vi "Actor Core.vi"(8 "error in":errorcluster, 11 "HIJ Vision Camera App Dialog in":refnum<class "HIJ Vision Camera App Dialog.lvclass">) -> (0 "error out":errorcluster, 3 "Actor out":refnum<class "Actor.lvclass">)   [LabVIEW 2014, in "HIJ Vision Camera App Dialog.lvlib" / "HIJ Vision Camera App Dialog.lvclass"]
doc: "(<B>Filename</B>: Actor Framework.lvlib:Actor.lvclass:Actor Core.vi)\n\nReceives messages to the actor, reacts to them, and initiates any error handling that may shut the actor down.\n\nDescendant classes may override this VI to append parallel tasks for the actor to complete while it handles messages. Overrides use the Call Parent Method node."
uses:
  HIJ Vision Camera App Dialog.lvclass
  <vilib>/ActorFramework/Actor/Actor.lvclass
  <vilib>/userdefined/High Color/IMAQdx.ctl
  Shared Code/Viewable Actor/ViewableActor/ViewableActor.lvclass/ViewableActor.ctl
  HIJ Vision Camera App Dialog.lvclass/HIJ Vision Camera App Dialog.ctl
  <vilib>/ActorFramework/Actor/Actor.lvclass/Actor.ctl
  <vilib>/ActorFramework/Message Enqueuer/Message Enqueuer.lvclass/Message Enqueuer.ctl
  HIJ Vision Camera App Dialog Messages/Update Data befor stop Msg/Update Data befor stop Msg.lvclass/Update Data befor stop Msg.ctl
  HIJ Vision Camera App/HIJ Vision Camera App Messages/Save Sequence Msg/Save Sequence Msg.lvclass/Save Sequence Msg.ctl
  HIJ Vision Application/HIJ Vision Application Messages/Write WorkDir Msg/Write WorkDir Msg.lvclass/Write WorkDir Msg.ctl
  HIJ Vision Camera App/HIJ Vision Camera App Messages/Write ConfigDir Msg/Write ConfigDir Msg.lvclass/Write ConfigDir Msg.ctl
  HIJ Vision Application/HIJ Vision Application Messages/Write Image Prefix Msg/Write Image Prefix Msg.lvclass/Write Image Prefix Msg.ctl
  HIJ Vision Camera App/HIJ Vision Camera App Messages/Start Aquisition Msg/Start Aquisition Msg.lvclass/Start Aquisition Msg.ctl
  HIJ Vision Camera App/HIJ Vision Camera App Messages/Change Camera Msg/Change Camera Msg.lvclass/Change Camera Msg.ctl
  Shared Code/Viewable Actor/ViewableActor/Write UI VI Ref.vi
  Read Camera Name.vi
  Read ConfigDir.vi
  Read Prefix.vi
  Read WorkDir.vi
  Read Acquire.vi
  <vilib>/ActorFramework/Message Enqueuer/Init from Existing Queue.vi
  <vilib>/ActorFramework/Message Enqueuer/Enqueue.vi
  <vilib>/ActorFramework/Message Priority Queue/Priority Enqueue.vi
  <vilib>/ActorFramework/Message Enqueuer/Message Enqueuer.lvclass
  HIJ Vision Camera App Dialog Messages/Update Data befor stop Msg/Update Data befor stop Msg.lvclass
  <vilib>/ActorFramework/Stop Msg/Stop Msg.lvclass
  HIJ Vision Camera App/HIJ Vision Camera App Messages/Save Sequence Msg/Save Sequence Msg.lvclass
  HIJ Vision Application/HIJ Vision Application Messages/Write WorkDir Msg/Write WorkDir Msg.lvclass
  HIJ Vision Camera App/HIJ Vision Camera App Messages/Write ConfigDir Msg/Write ConfigDir Msg.lvclass
  HIJ Vision Application/HIJ Vision Application Messages/Write Image Prefix Msg/Write Image Prefix Msg.lvclass
  HIJ Vision Camera App/HIJ Vision Camera App Messages/Stop Aquisition Msg/Stop Aquisition Msg.lvclass
  HIJ Vision Camera App/HIJ Vision Camera App Messages/Start Aquisition Msg/Start Aquisition Msg.lvclass
  HIJ Vision Camera App/HIJ Vision Camera App Messages/Change Camera Msg/Change Camera Msg.lvclass
  Shared Code/Viewable Actor/ViewableActor/ViewableActor.lvclass
panel:
  in  "Acquire":bool
  in  "stop":bool
  in  "Camera Name":T1="TestCam"
  in  "#to save":u16=10
  in  "Save Seq.":bool
  in  "Prefix":string
  out "Current Nr.":u16=10
  in  "WorkDir":path=path "C:/Users/user/Desktop/test/WorkDir"
  in  "ConfigDir":path=path "C:/Users/user/Desktop/test/ConfigDir"
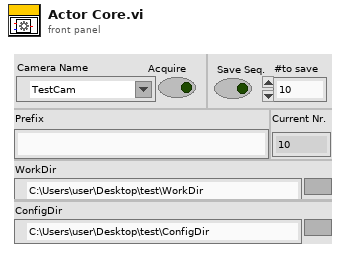
[diagram p1: front panel]
types:
  T1 = typedef "IMAQdx.ctl" = refnum<k21>
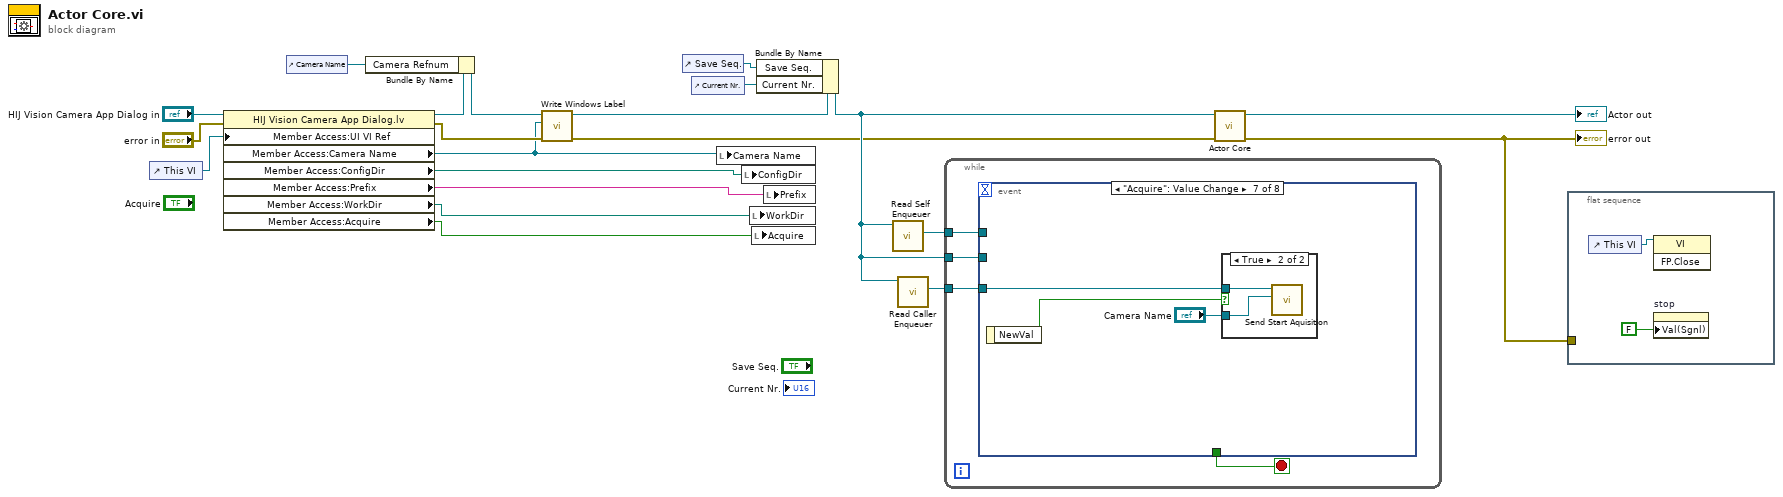
[diagram p0: block diagram]
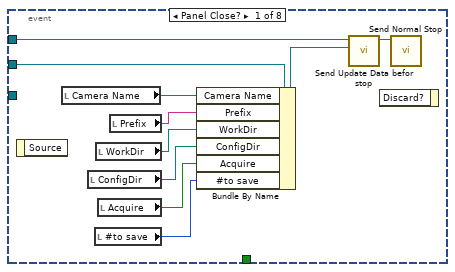
[diagram p2: hidden frame]
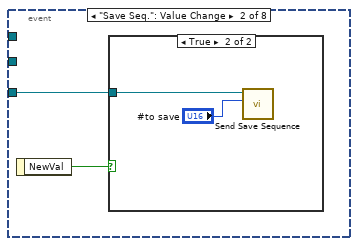
[diagram p3: hidden frame]
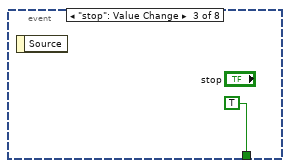
[diagram p5: hidden frame]
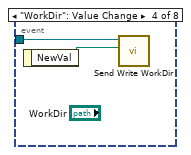
[diagram p6: hidden frame]
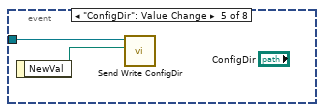
[diagram p7: hidden frame]
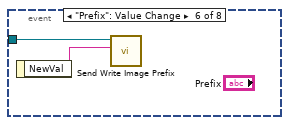
[diagram p8: hidden frame]
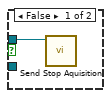
[diagram p9: hidden frame]
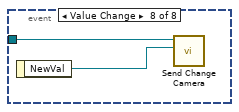
[diagram p10: hidden frame]
diagram:
  n1 = control-ref of="This VI"() -> (w17:refnum<vi>)
  n2 = property class="HIJ Vision Camera App Dialog.lv"(reference="HIJ Vision Camera App Dialog in", error in="error in", "Member Access:UI VI Ref"=w17) -> (reference out=w7:refnum<class "HIJ Vision Camera App Dialog.lvclass">, error out=w5:errorcluster, "Member Access:Camera Name"=w3:T1, "Member Access:ConfigDir"=w13:path, "Member Access:Prefix"=w12:string, "Member Access:WorkDir"=w14:path, "Member Access:Acquire"=w11:bool)
  n3 = control-ref of="Camera Name"() -> (w1:refnum<vi>)
  n4 = Bundle By Name(cluster=w7, "Camera Refnum"=w1) -> (w2:refnum<class "HIJ Vision Camera App Dialog.lvclass">)
  n5 = call-dynamic "Write Windows Label.vi"("error in (no error)"=w5, "Windows Label"=w3, "ViewableActor in"=w2) -> ("error out"=w4:errorcluster, "ViewableActor out"=w6:refnum<class "HIJ Vision Camera App Dialog.lvclass">)  [unwired: 7 in]
  n6 = control-ref of="Save Seq."() -> (w8:refnum<vi>)
  n7 = control-ref of="Current Nr."() -> (w9:refnum<vi>)
  n8 = local write "Camera Name"(w3) -> ()
  n9 = local write "ConfigDir"(w13) -> ()
  n10 = local write "WorkDir"(w14) -> ()
  n11 = local write "Acquire"(w11) -> ()
  n12 = Bundle By Name(cluster=w6, "Save Seq."=w8, "Current Nr."=w9) -> (w10:refnum<class "HIJ Vision Camera App Dialog.lvclass">)
  n13 = local write "Prefix"(w12) -> ()
  n14 = call <vilib>:"Read Self Enqueuer.vi"("Actor"=w10) -> ("Self Enqueuer"=w20:refnum<class "Message Enqueuer.lvclass">)  [unwired: 10 in]
  n15 = call <vilib>:"Read Caller Enqueuer.vi"("Actor"=w10) -> ("Caller Enqueuer"=w15:refnum<class "Message Enqueuer.lvclass">)  [unwired: 10 in]
  n16 = while {
    tunnel: w20 -> [w25]
    tunnel: w15 -> [w23]
    tunnel: w10 -> [w22]
    stop <- w24 stop-if-true
    n17 = event shown="[6] \"Acquire\": Value Change" {
      selector: _ -> [_ _ _ _ _ _ _ _]
      dyn-events: _ -> [_ _ _ _ _ _ _ _]
      timeout: _ -> [_ _ _ _ _ _ _ _]
      tunnel: w25 -> [w29 _ _ _ _ _ _ _]
      tunnel: [_ _ TRUE _ _ _ _ _] -> w24
      tunnel: w23 -> [_ w37 _ w42 w44 w46 w48 w54]
      tunnel: w22 -> [w35 _ _ _ _ _ _ _]
      event Panel Close? {
        n18 = event-data() -> ()  [unwired: 1 in, 1 out]
        n19 = local read "Camera Name"() -> (w34:T1)
        n20 = local read "ConfigDir"() -> (w32:path)
        n21 = local read "#to save"() -> (w26:u16)
        n22 = local read "WorkDir"() -> (w31:path)
        n23 = local read "Acquire"() -> (w30:bool)
        n24 = local read "Prefix"() -> (w33:string)
        n25 = Bundle By Name(cluster=w35, "Camera Name"=w34, "Prefix"=w33, "WorkDir"=w31, "ConfigDir"=w32, "Acquire"=w30, "#to save"=w26) -> (w27:refnum<class "HIJ Vision Camera App Dialog.lvclass">)
        n26 = call "Send Update Data befor stop.vi"("Current State"=w27, "Message Enqueuer"=w29) -> ("Message Enqueuer out"=w28:refnum<class "Message Enqueuer.lvclass">)  [unwired: 8 in, 1 out]
        n27 = event-data() -> ()  [unwired: 2 in, 1 out]
        n28 = call <vilib>:"Send Normal Stop.vi"("Message Enqueuer"=w28) -> ()  [unwired: 10 in, 1 out]
      }
      event "Save Seq.": Value Change {
        n29 = event-data() -> ("NewVal"=w36:bool)  [unwired: 1 in]
        n30 = case shown="True" w36 {
          tunnel: w37 -> [_ w38]
          frame False {
          }
          frame True {
            n31 = call "Send Save Sequence.vi"("#to save"="#to save", "Message Enqueuer"=w38) -> ()  [unwired: 8 in, 2 out]
          }
        }
      }
      event "stop": Value Change {
        n32 = event-data() -> ()  [unwired: 1 in, 1 out]
      }
      event "WorkDir": Value Change {
        n33 = event-data() -> ("NewVal"=w41:path)  [unwired: 1 in]
        n34 = call "Send Write WorkDir.vi"("Work Dir"=w41, "Message Enqueuer"=w42) -> ()  [unwired: 8 in, 2 out]
      }
      event "ConfigDir": Value Change {
        n35 = event-data() -> ("NewVal"=w43:path)  [unwired: 1 in]
        n36 = call "Send Write ConfigDir.vi"("Work Dir"=w43, "Message Enqueuer"=w44) -> ()  [unwired: 8 in, 2 out]
      }
      event "Prefix": Value Change {
        n37 = event-data() -> ("NewVal"=w45:string)  [unwired: 1 in]
        n38 = call "Send Write Image Prefix.vi"("Prefix"=w45, "Message Enqueuer"=w46) -> ()  [unwired: 8 in, 2 out]
      }
      event "Acquire": Value Change {
        n39 = event-data() -> ("NewVal"=w49:bool)  [unwired: 1 in]
        n40 = case shown="True" w49 {
          tunnel: w48 -> [w50 w52]
          tunnel: "Camera Name" -> [_ w51]
          frame False {
            n41 = call "Send Stop Aquisition.vi"("Message Enqueuer"=w50) -> ()  [unwired: 9 in, 2 out]
          }
          frame True {
            n42 = call "Send Start Aquisition.vi"("Camera"=w51, "Message Enqueuer"=w52) -> ()  [unwired: 8 in, 2 out]
          }
        }
      }
      event Value Change {
        n43 = event-data() -> ("NewVal"=w53:T1)  [unwired: 1 in]
        n44 = call "Send Change Camera.vi"("New Camera"=w53, "Message Enqueuer"=w54) -> ()  [unwired: 8 in, 2 out]
      }
    }
  }
  n45 = call-parent "Actor Core.vi"("error in"=w4, "Actor in"=w10) -> ("error out"=w19:errorcluster, "Actor out"=→"Actor out":refnum<class "Actor.lvclass">)  [unwired: 8 in]
  "error out" <- w19
  n46 = flat-sequence {
    tunnel: w19 -> [_]
    frame #0 {
      n47 = control-ref of="This VI"() -> (w55:refnum<vi>)
      n48 = invoke class="VI" method="FP.Close"(reference=w55) -> ()  [unwired: 2 in, 3 out]
      n49 = property on="stop" class="Bool (strict)"("Val(Sgnl)"=FALSE ("Value (Signaling)")) -> ()  [unwired: 2 in, 2 out]
    }
  }
